vi "test_serpenbot_DDPG_control.vi"() -> ()   [LabVIEW 2020]
panel:
  out "current y":dbl
  out "current x":dbl
  in  "goal y":dbl
  in  "goal x":dbl
  out "laser control value":dbl[](array[numeric])
  out "done":bool
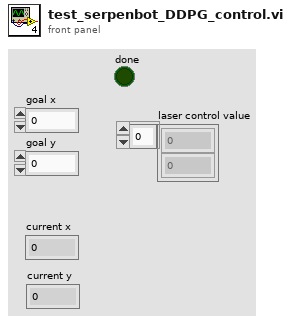
[diagram p1: front panel]
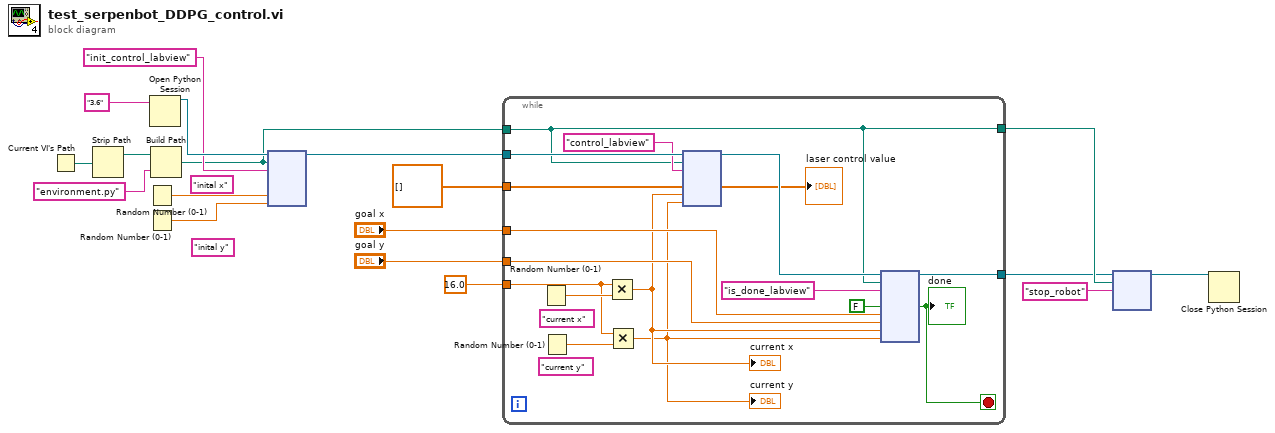
[diagram p0: block diagram]
diagram:
  (unwired) "inital y"
  (unwired) "inital x"
  n1 = Current VI's Path() -> (path=w18:path)
  n2 = Strip Path(path=w18) -> (stripped path=w17:path)  [unwired: 1 out]
  n3 = Random Number (0-1)() -> (number: 0 to 1=w12:dbl)
  n4 = Random Number (0-1)() -> (number: 0 to 1=w11:dbl)
  n5 = Open Python Session(python version="3.6" ("Python version")) -> (session out=w14:refnum<k35>)  [unwired: 2 in, 1 out]
  n6 = Build Path(base path=w17, name or relative path="environment.py") -> (appended path=w10:path)
  n7 = node(w14, w10, "init_control_labview" ("function name"), w12, w11) -> (w9:refnum<k35>)  [unwired: 5 in, 3 out]
  n8 = while {
    tunnel: w9 -> [w35]
    tunnel: [w29] -> w5
    tunnel: w10 -> [w21]
    tunnel: dbl[] [] -> [w28]
    tunnel: "goal x" -> [w24]
    tunnel: "goal y" -> [w23]
    tunnel: 16.0 -> [w22]
    tunnel: [w21] -> w6
    stop <- w30 stop-if-true
    (unwired) "current y"
    (unwired) "current x"
    n9 = Random Number (0-1)() -> (number: 0 to 1=w26:dbl)
    n10 = Random Number (0-1)() -> (number: 0 to 1=w25:dbl)
    n11 = Multiply(x=w22, y=w26) -> (x*y=w20:dbl)
    "current x" <- w20
    n12 = Multiply(x=w22, y=w25) -> (x*y=w19:dbl)
    "current y" <- w19
    n13 = node(w35, w21, "control_labview" ("function name"), w28, w20, w19) -> (w33:refnum<k35>, →"laser control value":dbl[])  [unwired: 3 in, 3 out]
    n14 = node(w33, w21, "is_done_labview" ("function name"), FALSE, w24, w23, w20, w19) -> (w29:refnum<k35>, w30:bool)  [unwired: 5 in, 3 out]
    "done" <- w30
  }
  n15 = node(w5, w6, "stop_robot" ("function name")) -> (w3:refnum<k35>)  [unwired: 3 in, 3 out]
  n16 = Close Python Session(session in=w3) -> ()  [unwired: 1 in, 1 out]
